vi "Set contrls enabled disabled.vi"(11 "error in (no error)":errorcluster) -> (15 "error out":errorcluster)   [LabVIEW 2011]
uses:
  Measurments Handling/Common/Variable List Common Digital.ctl
  Measurments Handling/Status Digitalish.ctl
  Controll refrence groups.ctl
  Application Structure/Options/Action GFV Settings.ctl
  Measurments Handling/Common/Variable List Common Analog.ctl
  emi Lib/Basic/1 - GUI/Control tools/Private/emi_Control enable and visibility array.vi
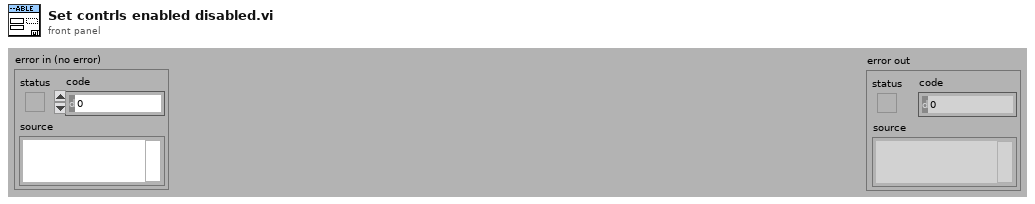
[diagram p1: front panel]
types:
  T1 = typedef "Variable List Common Analog.ctl" = enum16{"HVPSU Head Voltage", "HVPSU TS Voltage", "HVPSU Current", "PCP Cable Resistance", "Winch Depth", "Winch Line Speed", "Winch Wire Tension"}
  T2 = typedef "Action GFV Settings.ctl" = enum16{"Init", "Get From INI", "Put In INI", "Get Settings", "Get Update Index", "Set Setting"}
  T3 = typedef "Controll refrence groups.ctl" = enum16{"Controller. gen", "Controller . High G", "Stroker", "PCP Online", "PCP Local", "PCP HV On", "Driller", "Stroker Cmd Buttons", "Stroker Anchor Cmd Buttons", "Controller Relay Buttons", "PCP Start Telemetry", "PCP Start Motor", "Tractor", "Modem Status"}
  T4 = typedef "Status Digitalish.ctl" = enum16{"NA", "False", "True"}
  T5 = typedef "Variable List Common Digital.ctl" = enum16{"PCP Connected", "PCP PC Control", "HV PSU connected", "HV PSU HV Active", "Modem Connected", "Tool Connected", "CanBus interface"}
  T6 = typedef "Options  All pages and custom.ctl" = cluster{"P 1 (App)":T7, "P 2":T8, "P 3":T9, "P 4":T12, "P 5":T17, "P 6 (Err)":T18, "P 7 (Expert)":T19, "P 8 (Depth)":T21, "C 1":T22, "C 2":T23}
  T7 = typedef "Options Page 1 (App).ctl" = cluster{"Result files":path, "PCP Interface":string, "Tractor/Stroker Interface":string, "Tractor Interface":string, "Modem Status Interface":string, "Audible Alarm":bool, "Force alarm on Technical":bool, "Force alarm on HH":bool, "Force alarm on LL":bool, "Force alarm on H":bool, "Force alarm on L":bool}
  T8 = typedef "Options Page 2.ctl" = cluster{"Solenoid & Relay latching time":u16, "Tractor relay 1":dbl, "Tractor relay 2":dbl, "Tractor Solenoid limit":dbl}
  T9 = typedef "Options Page 3.ctl" = cluster{"Min resistance":dbl, "Max resistance":dbl, "Head voltage range":T10, "Max voltage jump":dbl, "Maximum resistance change":dbl, "Start Telemetry Voltage":dbl, "Start Telemetry Timeout":dbl, "Start Motor Voltage":dbl, "Stop Motor Voltage":dbl, "Pass Mode Warning Voltage":dbl, "Relay Switch Voltage":dbl, "Relay Status Loss Voltage":dbl, "Samples to average":i32, "PSU type DO NOT USE":T11, "Magna OVP":dbl, "Magna Current Limit":dbl}
  T10 = typedef "PCP type List.ctl" = enum16{"0 - 350V", "0 - 450V", "0 - 600V"}
  T11 = typedef "PSU Type.ctl" = enum16{"Unipower", "Magna 8.3A", "Magna 12A", "None"}
  T12 = typedef "Options Page 4.ctl" = cluster{"Solenoid & Relay latching time":u16, "Stroker relay 1":dbl, "Stroker Relay 2":dbl, "Stroker Solenoid limit":dbl, "Force det.":T13, "Stroke force lim.":dbl, "Anchor Enabled Pressure":dbl, "Tacometer puls":dbl, "Default anchor behavior":T14, "Default stroker behavior":T15, "Default stroker force limit (tonne)":dbl, "Slips Size":T16}
  T13 = typedef "Stroke force selector.ctl" = enum16{"Stroke in = node 1", "Strok out = node 1"}
  T14 = typedef "Default anchor behavior.ctl" = enum16{"Do nothing", "Set Anchor", "Release Anchor"}
  T15 = typedef "Default stroker behavior.ctl" = enum16{"Do nothing", "Stop", "Go Out", "Go In"}
  T16 = typedef "Slips Type Radio.ctl" = enum32{"No Selection", "338 MRS", "3,9 MRS"}
  T17 = typedef "Options Page 5.ctl" = cluster{"Solenoid & Relay latching time":u16, "Driller relay 1":dbl, "Driller Relay 2":dbl, "Driller  Solenoid limit":dbl}
  T18 = typedef "Options Page 6 (Err).ctl" = cluster{"Error and event files":path}
  T19 = typedef "Options Page 7 (Expert).ctl" = cluster{"Show Debug":bool, "Log debug messages":bool, "Additional debug messages":bool, "Start Beagle with Simulator data":bool, "Workshop mode":bool, "Modem baud":u16, "enumCANCOM":bool, "Modem sim":T20, "Telemetry Timeout Disable":i32, "Buffer size":i32, "Upd regular data":bool, "Cable comp":cluster{"VMOD1 Voltage(V)":dbl, "VMOD2 Voltage(V)":dbl}}
  T20 = typedef "Modem simulation setup.ctl" = cluster{"Modem dealay sim":bool, "Sim baud Tx":u16, "Bit Error fraction Tx":dbl, "Sim baud Rx":u16, "Bit Error fraction Rx":dbl}
  T21 = typedef "Options Page 8 (Depth).ctl" = cluster{"Winch Spool Circumference":dbl, "Winch Pulses per Revolution":dbl, "Current Depth":dbl}
  T22 = typedef "Options Custom 1.ctl" = cluster{"Depth Updated":bool, "Depth Offset":dbl}
  T23 = typedef "Options Custom 2.ctl" = cluster{"Placeholder":bool}
  T24 = cluster{"Controll collection":T3, bool, "State(Normal)":enum16{"Normal", "Disabled", "Grayed", "Hidden"}}
  T25 = cluster{"Controll collection":T3, bool, "State(Normal)":enum16{"Normal", "Disabled", "Grayed", "Hidden"}}[]
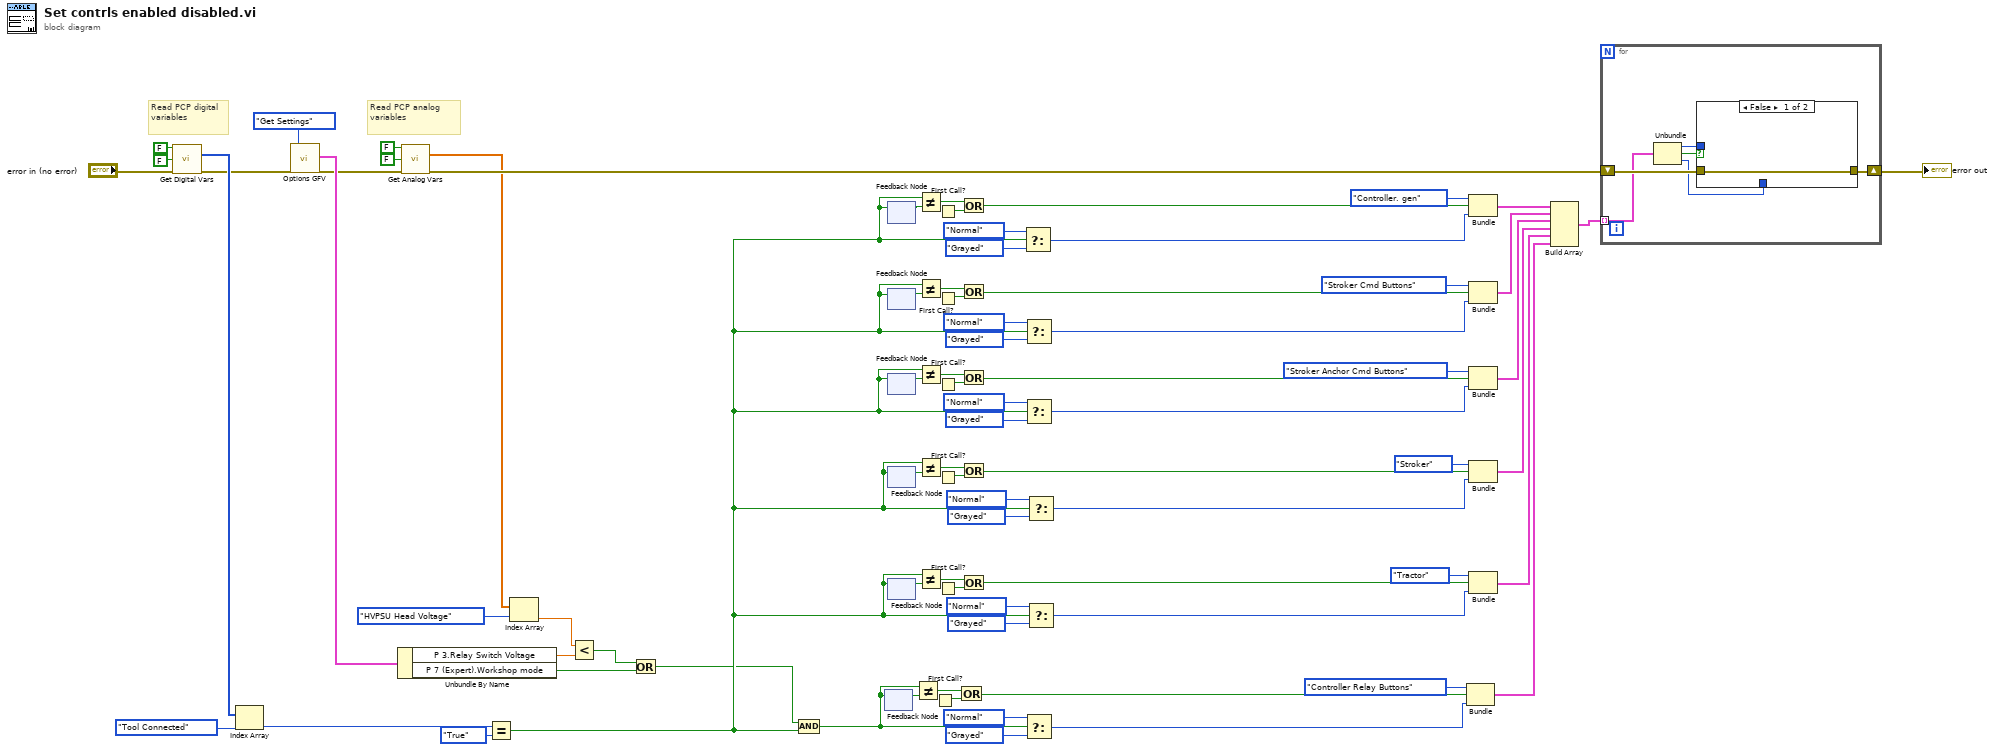
[diagram p0: block diagram]
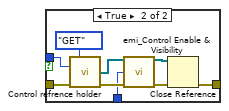
[diagram p2: hidden frame]
diagram:
  # "Read PCP analog variables"
  # "Read PCP digital variables"
  n1 = call "Get Digital Vars.vi"("Common alarm handling(F)"=FALSE, "Tool"=FALSE, "error in (no error)"="error in (no error)") -> ("Values"=w43:T4[], "error out"=w8:errorcluster)  [unwired: 6 in, 5 out]
  n2 = Index Array(array=w43, index=Variable_List_Common_Digital."Tool Connected" ("Action")) -> (element=w40:T4)
  n3 = call "Options GFV.vi"("error in (no error)"=w8, "Action(Get Settings)"=Action_GFV_Settings."Get Settings") -> ("Options"=w12:T6, "error out"=w7:errorcluster)  [unwired: 15 in, 1 out]
  n4 = Unbundle By Name(w12) -> ("P 3.Relay Switch Voltage"=w14:dbl, "P 7 (Expert).Workshop mode"=w16:bool)
  n5 = call "Get Analog Vars.vi"("Common alarm handling(F)"=FALSE, "Tool"=FALSE, "error in (no error)"=w7) -> ("Values"=w6:dbl[], "error out"=w9:errorcluster)  [unwired: 6 in, 5 out]
  n6 = Equal?(x=w40, y=Status_Digitalish."True") -> (x = y?=w3:bool)
  n7 = Index Array(array=w6, index=Variable_List_Common_Analog."HVPSU Head Voltage" ("First part list")) -> (element=w5:dbl)
  n8 = Less?(x=w5, y=w14) -> (x < y?=w15:bool)
  n9 = Or(x=w15, y=w16) -> (x .or. y?=w1:bool)
  n10 = Compound Arithmetic op=AND(w1, w3) -> (w2:bool)
  n11 = feedback #1() -> (w23:bool)  [unwired: 1 in]
  n12 = feedback-in #1(w2) -> ()
  n13 = feedback #2() -> (w44:bool)  [unwired: 1 in]
  n14 = feedback-in #2(w3) -> ()
  n15 = feedback #3() -> (w49:bool)  [unwired: 1 in]
  n16 = feedback-in #3(w3) -> ()
  n17 = feedback #4() -> (w50:bool)  [unwired: 1 in]
  n18 = feedback-in #4(w3) -> ()
  n19 = feedback #5() -> (w55:bool)  [unwired: 1 in]
  n20 = feedback-in #5(w3) -> ()
  n21 = feedback #6() -> (w56:bool)  [unwired: 1 in]
  n22 = feedback-in #6(w3) -> ()
  n23 = Not Equal?(x=w2, y=w23) -> (x != y?=w21:bool)
  n24 = Not Equal?(x=w3, y=w44) -> (x != y?=w46:bool)
  n25 = Not Equal?(x=w3, y=w49) -> (x != y?=w47:bool)
  n26 = Not Equal?(x=w3, y=w50) -> (x != y?=w52:bool)
  n27 = Not Equal?(x=w3, y=w55) -> (x != y?=w53:bool)
  n28 = Not Equal?(x=w3, y=w56) -> (x != y?=w58:bool)
  n29 = First Call?() -> (First Call?: T/F=w22:bool)
  n30 = First Call?() -> (First Call?: T/F=w45:bool)
  n31 = First Call?() -> (First Call?: T/F=w48:bool)
  n32 = First Call?() -> (First Call?: T/F=w51:bool)
  n33 = First Call?() -> (First Call?: T/F=w54:bool)
  n34 = First Call?() -> (First Call?: T/F=w57:bool)
  n35 = Or(x=w21, y=w22) -> (x .or. y?=w19:bool)
  n36 = Or(x=w46, y=w45) -> (x .or. y?=w59:bool)
  n37 = Or(x=w47, y=w48) -> (x .or. y?=w68:bool)
  n38 = Or(x=w52, y=w51) -> (x .or. y?=w70:bool)
  n39 = Or(x=w53, y=w54) -> (x .or. y?=w72:bool)
  n40 = Or(x=w58, y=w57) -> (x .or. y?=w74:bool)
  n41 = Select(t=enum16{"Normal", "Disabled", "Grayed", "Hidden"}."Normal" ("State(Normal)"), s=w3, f=enum16{"Normal", "Disabled", "Grayed", "Hidden"}."Grayed" ("State(Normal)")) -> (s? t:f=w61:enum16{"Normal", "Disabled", "Grayed", "Hidden"})
  n42 = Select(t=enum16{"Normal", "Disabled", "Grayed", "Hidden"}."Normal" ("State(Normal)"), s=w3, f=enum16{"Normal", "Disabled", "Grayed", "Hidden"}."Grayed" ("State(Normal)")) -> (s? t:f=w69:enum16{"Normal", "Disabled", "Grayed", "Hidden"})
  n43 = Select(t=enum16{"Normal", "Disabled", "Grayed", "Hidden"}."Normal" ("State(Normal)"), s=w3, f=enum16{"Normal", "Disabled", "Grayed", "Hidden"}."Grayed" ("State(Normal)")) -> (s? t:f=w71:enum16{"Normal", "Disabled", "Grayed", "Hidden"})
  n44 = Select(t=enum16{"Normal", "Disabled", "Grayed", "Hidden"}."Normal" ("State(Normal)"), s=w2, f=enum16{"Normal", "Disabled", "Grayed", "Hidden"}."Grayed" ("State(Normal)")) -> (s? t:f=w18:enum16{"Normal", "Disabled", "Grayed", "Hidden"})
  n45 = Select(t=enum16{"Normal", "Disabled", "Grayed", "Hidden"}."Normal" ("State(Normal)"), s=w3, f=enum16{"Normal", "Disabled", "Grayed", "Hidden"}."Grayed" ("State(Normal)")) -> (s? t:f=w73:enum16{"Normal", "Disabled", "Grayed", "Hidden"})
  n46 = Select(t=enum16{"Normal", "Disabled", "Grayed", "Hidden"}."Normal" ("State(Normal)"), s=w3, f=enum16{"Normal", "Disabled", "Grayed", "Hidden"}."Grayed" ("State(Normal)")) -> (s? t:f=w75:enum16{"Normal", "Disabled", "Grayed", "Hidden"})
  n47 = Bundle("Controll collection"=Controll_refrence_groups."Controller Relay Buttons", w19, "State(Normal)"=w18) -> (w17:T24)  [unwired: 1 in]
  n48 = Bundle("Controll collection"=Controll_refrence_groups."Controller. gen", w59, "State(Normal)"=w61) -> (w66:T24)  [unwired: 1 in]
  n49 = Bundle("Controll collection"=Controll_refrence_groups."Stroker Cmd Buttons", w68, "State(Normal)"=w69) -> (w76:T24)  [unwired: 1 in]
  n50 = Bundle("Controll collection"=Controll_refrence_groups."Stroker Anchor Cmd Buttons", w70, "State(Normal)"=w71) -> (w77:T24)  [unwired: 1 in]
  n51 = Bundle("Controll collection"=Controll_refrence_groups."Stroker", w72, "State(Normal)"=w73) -> (w78:T24)  [unwired: 1 in]
  n52 = Bundle("Controll collection"=Controll_refrence_groups."Tractor", w74, "State(Normal)"=w75) -> (w79:T24)  [unwired: 1 in]
  n53 = Build Array(w66, w76, w77, w78, w79, w17) -> (w67:T25)
  n54 = for {
    tunnel: w67 -> [w84] mode=indexing
    shift-right: [w80] -> w27
    shift-left: w9 -> [w85]
    n55 = Unbundle(w84) -> ("Controll collection"=w83:T3, w82:bool, "State(Normal)"=w81:enum16{"Normal", "Disabled", "Grayed", "Hidden"})
    n56 = case shown="False" w82 {
      tunnel: w85 -> [w86 w91]
      tunnel: [w86 w90] -> w80
      tunnel: w83 -> [_ w89]
      tunnel: w81 -> [_ w88]
      frame False {
      }
      frame True {
        n57 = call "Control refrence holder.vi"("Action(GET)"=enum16{"GET", "SET"}."GET", "Controll collection"=w89, "error in (no error)"=w91) -> ("Controlls out"=w95:refnum<vi>[], "error out"=w94:errorcluster)  [unwired: 11 in]
        n58 = call-poly "emi_Control Enable & Visibility.vi"("Controls"=w95, "State(Normal)"=w88, "error in"=w94) -> ("Constrols out"=w92:refnum<vi>[], "error out"=w93:errorcluster)  [unwired: 11 in]
        n59 = Close Reference(reference=w92, error in (no error)=w93) -> (error out=w90:errorcluster)
      }
    }
  }
  "error out" <- w27
